vi "ASC码数字转化为数字.vi"(2 "字节数":u8=4, 3 "输入ASC码":string) -> (0 "输出字符串":string)   [LabVIEW 2009]
panel:
  # "如“192”-》192-》“C0”"
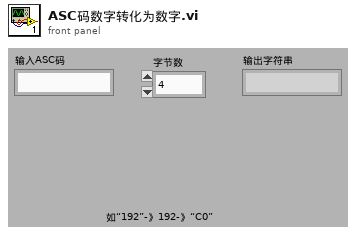
[diagram p1: front panel]
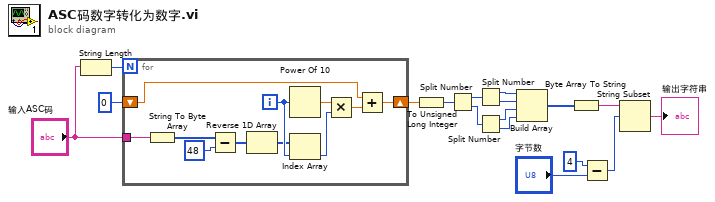
[diagram p0: block diagram]
diagram:
  n1 = String Length(string="输入ASC码") -> (length=w16:i32)
  n2 = for {
    N: w16 -> [_]
    tunnel: "输入ASC码" -> [w28]
    shift-right: [w25] -> w14
    shift-left: 0 -> [w24]
    i -> [w21]
    n3 = String To Byte Array(string=w28) -> (unsigned byte array=w27:u8[])
    n4 = Subtract(x=w27, y=48) -> (x-y=w19:i32[])
    n5 = Reverse 1D Array(array=w19) -> (reversed array=w20:i32[])
    n6 = Power Of 10(x=w21) -> (10^x=w22:dbl)
    n7 = Index Array(array=w20, index=w21) -> (element=w18:i32)
    n8 = Multiply(x=w22, y=w18) -> (x*y=w23:dbl)
    n9 = Add(x=w24, y=w23) -> (x+y=w25:dbl)
  }
  n10 = To Unsigned Long Integer(number=w14) -> (unsigned 32bit integer=w10:u32)
  n11 = Split Number(x=w10) -> (hi(x)=w12:u16, lo(x)=w11:u16)
  n12 = Split Number(x=w12) -> (hi(x)=w6:u8, lo(x)=w5:u8)
  n13 = Split Number(x=w11) -> (hi(x)=w4:u8, lo(x)=w3:u8)
  n14 = Build Array(w6, w5, w4, w3) -> (w2:u8[])
  n15 = Byte Array To String(unsigned byte array=w2) -> (string=w1:string)
  n16 = Subtract(x=u8 4, y="字节数") -> (x-y=w8:u8)
  n17 = String Subset(string=w1, offset (0)=w8) -> (substring=→"输出字符串":string)  [unwired: 1 in]
